vi "Timeout.vi"(8 "error in (no error)":errorcluster, 9 "Timeout (ms)":i32=5000, 10 "Start Time":u32) -> (0 "error out":errorcluster, 4 "Timeout?":bool)   [LabVIEW 2011, in "LVH-KinectOne.lvlib"]
uses:
  LVH-KinectOne.lvlib
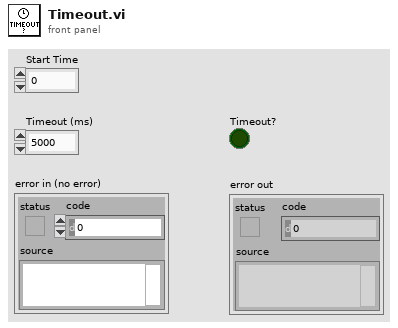
[diagram p1: front panel]
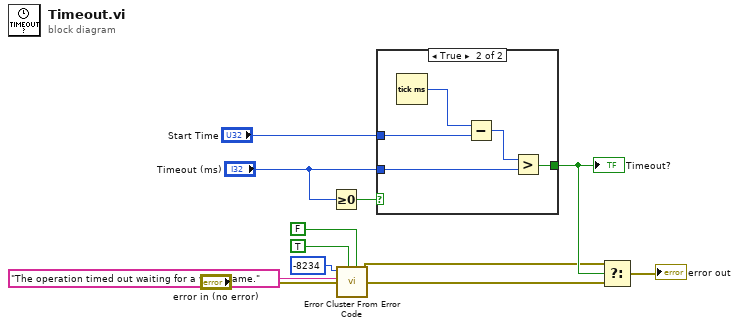
[diagram p0: block diagram]
diagram:
  n1 = Greater Or Equal To 0?(x="Timeout (ms)") -> (x >= 0?=w11:bool)
  n2 = call <vilib>:"Error Cluster From Error Code.vi"("is warning? (False)"=FALSE, "show call chain? (False)"=TRUE, "error message (\"\")"="The operation timed out waiting for a valid frame." ("error message (\"\")"), "error code (0)"=-8234) -> ("error out"=w7:errorcluster)  [unwired: 5 in]
  n3 = case shown="True" w11 {
    tunnel: "Timeout (ms)" -> [_ w13]
    tunnel: "Start Time" -> [_ w15]
    tunnel: [_ w12] -> w8
    frame False {
    }
    frame True {
      n4 = Tick Count (ms)() -> (millisecond timer value=w16:u32)
      n5 = Subtract(x=w16, y=w15) -> (x-y=w14:u32)
      n6 = Greater?(x=w14, y=w13) -> (0:w12:bool)
    }
  }
  "Timeout?" <- w8
  n7 = Select(t=w7, s=w8, f="error in (no error)") -> (s? t:f=→"error out":errorcluster)
